vi "TEST - Save VI ConPane Image.vi"(8 "error in (no error)":errorcluster) -> (0 "error out":errorcluster, 2 "pass":bool)   [LabVIEW 2009]
uses:
  <userlib>/_OpenG.lib/file/file.llb/Convert File Extension (Path)__ogtk.vi
panel:
  in  "new picture":picture
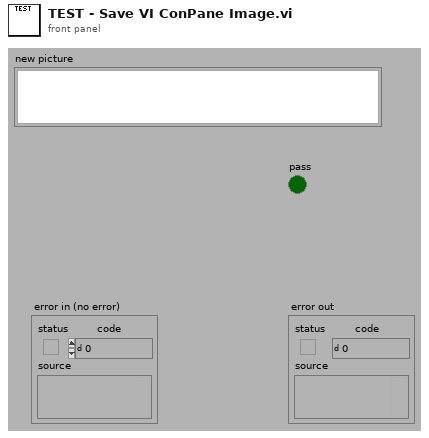
[diagram p1: front panel]
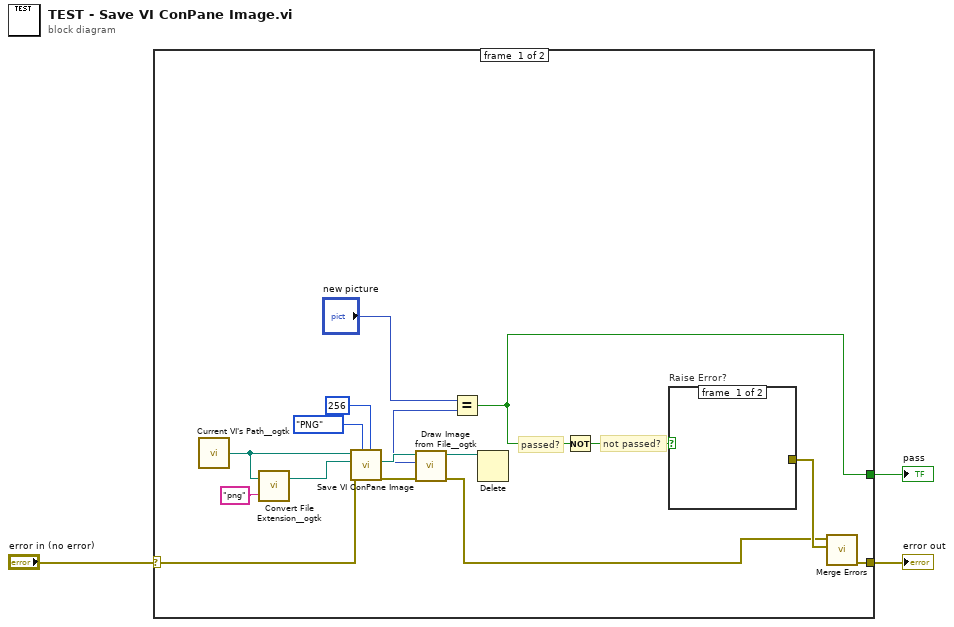
[diagram p0: block diagram]
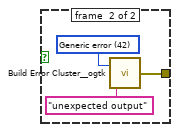
[diagram p2: hidden frame]
diagram:
  n1 = case shown="No Error" "error in (no error)" {
    selector: "error in (no error)" -> [w10 w22]
    tunnel: [w6 _] -> w3
    tunnel: [w18 w22] -> w1
    frame #0 {
      # "not passed?"
      # "passed?"
      n2 = call <userlib>:"Current VI's Path__ogtk.vi"() -> ("Current VI's Path (+ Relative)"=w13:path)  [unwired: 1 in]
      n3 = call-poly <userlib>:"Convert File Extension__ogtk.vi"("new ending (none)"="png", "file name"=w13) -> ("new filename"=w11:path)  [unwired: 1 out]
      n4 = call "Save VI ConPane Image.vi"("Image Depth (256)"=256 ("Image Depth"), "Image Format"=enum32{"PNG", "JPEG", "GIF"}."PNG", "error in (no error)"=w10, "Image File Path"=w11, "VI Path"=w13) -> ("error out"=w9:errorcluster)  [unwired: 6 in]
      n5 = call <userlib>:"Draw Image from File__ogtk.vi"("error in (no error)"=w9, "path to image file"=w11) -> ("error out"=w8:errorcluster, "new picture"=w5:picture, "dup path"=w7:path)  [unwired: 6 in, 1 out]
      n6 = Equal?(x="new picture", y=w5) -> (x = y?=w6:bool)
      n7 = Delete(path (use dialog)=w7) -> ()  [unwired: 4 in, 3 out]
      n8 = Not(x=w6) -> (.not. x?=w16:bool)
      n9 = case "Raise Error?" shown="True" w16 {
        tunnel: [_ w19] -> w17
        frame #0 {
        }
        frame #1 {
          w20 = 42 items=["No error", "Argument error", "Memory is full", "Out of zone", "End of file", "File already open", "Generic file I/O error", "File not found", "File permission error", "Disk is full", "Duplicate path", "Too many files open", "System feature not enabled", "Resource file not found", "Cannot add resource", "Resource not found", "Image not found", "Image memory error", "Pen does not exist", "Config type invalid", "Config token not found", "Config parse error", "Config memory error", "Bad external code format", "Bad external code offset", "External code not present", "Null window", "Destroy window error", "Null menu", "Print aborted", "Bad print record", "Print driver error", "Windows error during printing", "Memory error during printing", "Print dialog error", "Generic print error", "Invalid device refnum", "Device not found", "Device parameter error", "Device unit error", "Cannot open device", "Device call aborted", "Generic error", "Cancelled by user", "Object ID too low", "Object ID too high", "Object not in heap", "Unknown heap", "Unknown object (invalid DefProc)", "Unknown object (DefProc not in table)", "Message out of range", "Invalid (null) method", "Unknown message", "Manager call not supported", "Bad address", "Network operation in progress", "Network operation timed out", "Connection is busy", "Network attribute not supported", "Network error", "Address in use", "System out of memory", "Connection aborted", "Connection refused", "Not connected", "Already connected", "Connection closed", "Initialization error (interapplication manager)", "Bad occurrence", "Wait on unbound occurrence handler", "Occurrence queue overflow", "Datalog type conflict", "Unused", "Unrecognized type (interapplication manager)", "Memory corrupt", "Failed to make temporary DLL", "Old CIN version", "Drag socket not found", "Failed to load drop-object", "Failed to register OLE object", "Failed to release OLE object", "Format specifier type mismatch", "Unknown format specifier", "Too few format specifiers", "Too many format specifiers", "Scan failed", "Newer CIN version", "Error converting to variant", "Runtime menu error", "Password tampered", "Variant attribute not found", "Incompatible variant data type", "Event data is not available", "Event Store is not present", "Occurrence is not found", "Event Queue is not created", "Event info is not available", "Refnum passed is NULL", "Error retrieving Class GUID", "Error retrieving CoClass GUID", "Error retrieving TypeLib GUID.", "Bad built application magic bytes.", "Specific driver is different from the specific driver associated with the Logical Name.", "There is no session opened to the class driver.", "Max Error", "MAX - Error with config objects", "MAX - Error loading configuration", "MAX - Group not supported"]
          n10 = call <userlib>:"Build Error Cluster__ogtk.vi"("String to Prepend to source (\"\")"="unexpected output" ("String to Prepend to source (\"\")"), "code"=w20) -> ("error out"=w19:errorcluster)
        }
      }
      n11 = call <vilib>:"Merge Errors.vi"("error in 2 (no error)"=w17, "error in 1 (no error)"=w8) -> ("error out"=w18:errorcluster)  [unwired: 5 in]
    }
    frame #1 {
    }
  }
  "pass" <- w3
  "error out" <- w1
